vi "Build Error Message.vi"(8 "error in (no error)":errorcluster, 10 "Data":variant, 11 "Arg":string) -> (0 "error out":errorcluster)   [LabVIEW 2023, in "VI Properties Editor.lvlib" / "FaKI State Machine.lvlib"]
doc: "Appends text to the end of the error message indicating the State/Arg where the error occurred, and works in conjunction with <B>Producer Loop Guard Clause.vi</B> to catch and handle any errors that may have occurred in the Producer Loop."
uses:
  FaKI State Machine.lvlib
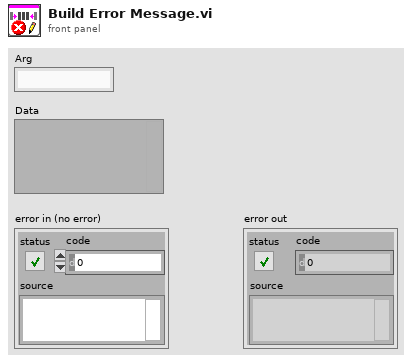
[diagram p1: front panel]
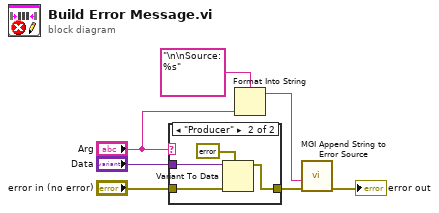
[diagram p0: block diagram]
diagram:
  n1 = case shown="\"Producer\"" "Arg" {
    tunnel: "Data" -> [_ w11]
    tunnel: "error in (no error)" -> [w8 w12]
    tunnel: [w8 w9] -> w5
    frame "", Default {
    }
    frame "Producer" {
      n2 = Variant To Data(error in=w12, type=errorcluster {"status"=FALSE, "code"=0, "source"=""} ("error out"), Variant=w11) -> (data=w9:errorcluster)  [unwired: 1 out]
    }
  }
  n3 = Format Into String(format string="\n\nSource: %s", "Arg") -> (resulting string=w2:string)  [unwired: 2 in, 1 out]
  n4 = call <userlib>:"MGI Append String to Error Source.vi"("Error In"=w5, "String to Append"=w2) -> ("Error Out"=→"error out":errorcluster)  [unwired: 9 in]
